vi "Calculate Index Array.vi"(8 "error in (no error)":errorcluster, 10 "3D Waterfall Datatype.lvclass in":refnum<class "3D Waterfall Datatype.lvclass">, 11 "Plot Representation In":T1) -> (0 "error out":errorcluster, 2 "3D Waterfall Datatype.lvclass out":refnum<class "3D Waterfall Datatype.lvclass">, 3 "Plot Representation Out":T1)   [LabVIEW 2017, in "3D Waterfall Datatype.lvclass"]
uses:
  <vilib>/Math Plots/3D Math Plots/3D Waterfall/3D Waterfall Datatype/3D Waterfall Datatype.lvclass
  <vilib>/Math Plots/3D Math Plots/3D Plot/3D Plot/Typedef/Plot Representation.ctl
  <vilib>/Math Plots/3D Math Plots/3D Plot/3D Plot/Typedef/Range Clusters.ctl
  <vilib>/Math Plots/3D Math Plots/3D Plot/3D Plot/Typedef/Mesh Data.ctl
  <vilib>/Math Plots/3D Math Plots/3D Plot/3D Plot/3D Plot.lvclass
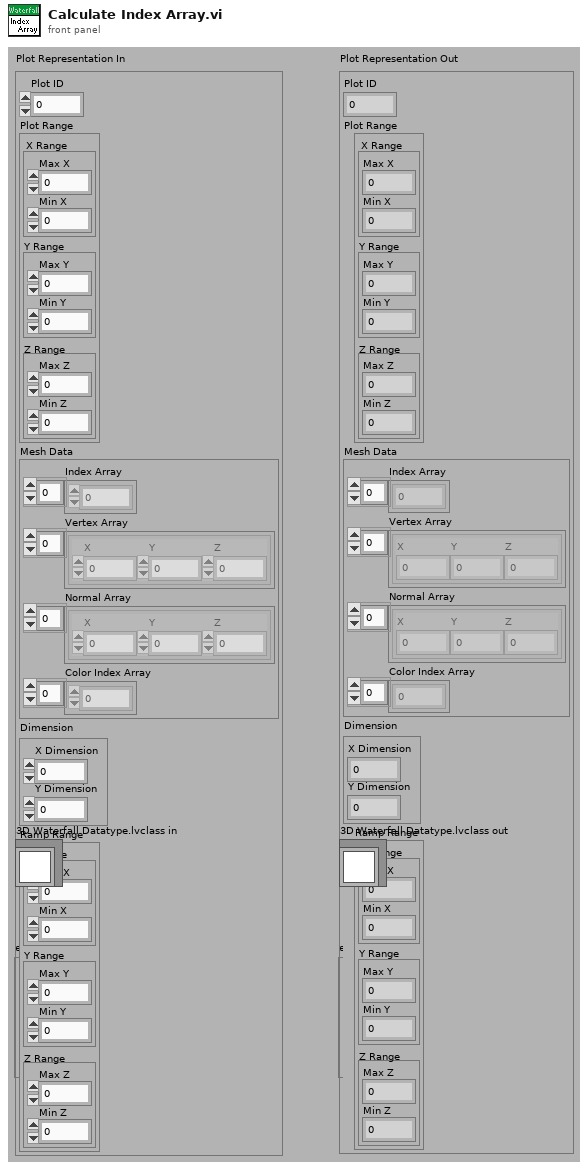
[diagram p1: front panel]
types:
  T1 = typedef "3D Plot.lvclass/Plot Representation.ctl" = cluster{"Plot ID":i32, "Plot Range":T2, "Mesh Data":T3, "Dimension":cluster{"X Dimension":i32, "Y Dimension":i32}, "Ramp Range":T2}
  T2 = typedef "3D Plot.lvclass/Range Clusters.ctl" = cluster{"X Range":cluster{"Max X":sgl, "Min X":sgl}, "Y Range":cluster{"Max Y":sgl, "Min Y":sgl}, "Z Range":cluster{"Max Z":sgl, "Min Z":sgl}}
  T3 = typedef "3D Plot.lvclass/Mesh Data.ctl" = cluster{"Index Array":u32[], "Vertex Array":cluster{"X":sgl, "Y":sgl, "Z":sgl}[], "Normal Array":cluster{"X":sgl, "Y":sgl, "Z":sgl}[], "Color Index Array":i32[]}
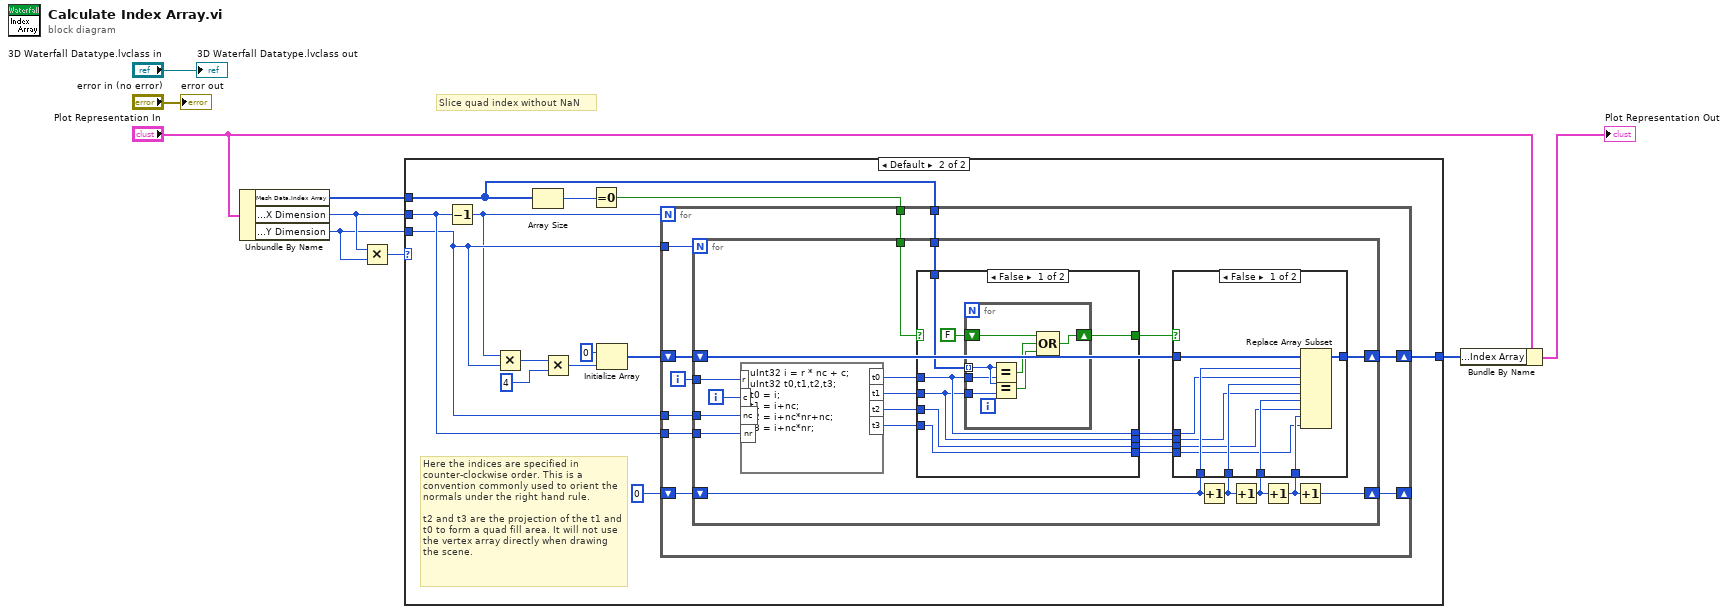
[diagram p0: block diagram]
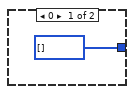
[diagram p2: hidden frame]
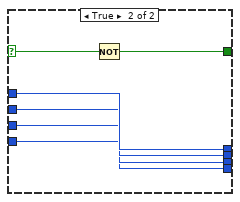
[diagram p4: hidden frame]
diagram:
  # "Slice quad index without NaN"
  n1 = Unbundle By Name("Plot Representation In") -> ("Mesh Data.Index Array"=w1:u32[], "Dimension.X Dimension"=w4:i32, "Dimension.Y Dimension"=w3:i32)
  n2 = Multiply(x=w4, y=w3) -> (x*y=w2:i32)
  n3 = case shown="Default" w2 {
    tunnel: [u32[] [] w23] -> w5
    tunnel: w4 -> [_ w17]
    tunnel: w3 -> [_ w16]
    tunnel: w1 -> [_ w12]
    frame 0 {
    }
    frame Default {
      # "Here the indices are specified in counter-clockwise order. This is a convention commonly used to orient the normals under the right hand rule.\n\nt2 and t3 are the projection of the t1 and t0 to form a quad fill area. It will not use the vertex array directly when drawing the scene."
      n4 = Decrement(x=w17) -> (x-1=w14:i32)
      n5 = Multiply(x=w14, y=w16) -> (x*y=w20:i32)
      n6 = Array Size(array=w12) -> (size(s)=w13:i32)
      n7 = Multiply(x=w20, y=4) -> (x*y=w22:i32)
      n8 = Equal To 0?(x=w13) -> (x = 0?=w11:bool)
      n9 = Initialize Array(u32 0, w22) -> (w18:u32[])
      n10 = for {
        N: w14 -> [_]
        shift-right: [w29] -> w23
        shift-left: w18 -> [w33]
        tunnel: w16 -> [w31]
        tunnel: w16 -> [w30]
        tunnel: w17 -> [w28]
        shift-right: [w27] -> _
        shift-left: 0 -> [w26]
        tunnel: w12 -> [w25]
        tunnel: w11 -> [w24]
        i -> [w32]
        n11 = for {
          N: w31 -> [_]
          tunnel: w32 -> [w55]
          tunnel: w30 -> [w53]
          shift-right: [w49] -> w29
          shift-left: w33 -> [w50]
          tunnel: w28 -> [w52]
          shift-right: [w51] -> w27
          shift-left: w26 -> [w45]
          tunnel: w25 -> [w44]
          tunnel: w24 -> [w43]
          i -> [w54]
          n12 = formula code="uInt32 i = r * nc + c; \nuInt32 t0,t1,t2,t3;\nt0 = i; \nt1 = i+nc; \nt2 = i+nc*nr+nc; \nt3 = i+nc*nr;"("r"=w55, "nc"=w53, "c"=w54, "nr"=w52) -> ("t0"=w42:u32, "t1"=w41:u32, "t2"=w40:u32, "t3"=w39:u32)
          n13 = case shown="False" w43 {
            selector: w43 -> [_ w82]
            tunnel: [w70 w86] -> w38
            tunnel: w42 -> [w70 w86]
            tunnel: [w69 w85] -> w37
            tunnel: w41 -> [w69 w85]
            tunnel: [w68 w84] -> w36
            tunnel: w40 -> [w68 w84]
            tunnel: [w67 w83] -> w35
            tunnel: w39 -> [w67 w83]
            tunnel: w44 -> [w73 _]
            tunnel: [w71 w81] -> w34
            frame False {
              n14 = for {
                tunnel: w73 -> [w80] mode=indexing
                tunnel: w70 -> [w79]
                tunnel: w69 -> [w74]
                shift-right: [w76] -> w71
                shift-left: FALSE -> [w75]
                n15 = Equal?(x=w80, y=w79) -> (x = y?=w78:bool)
                n16 = Equal?(x=w80, y=w74) -> (x = y?=w77:bool)
                n17 = Compound Arithmetic op=OR(w75, w78, w77) -> (w76:bool)
              }
            }
            frame True {
              n18 = Not(x=w82) -> (.not. x?=w81:bool)
            }
          }
          n19 = Increment(x=w45) -> (x+1=w46:i32)
          n20 = Increment(x=w46) -> (x+1=w47:i32)
          n21 = Increment(x=w47) -> (x+1=w48:i32)
          n22 = case shown="False" w34 {
            tunnel: w50 -> [w65 w66]
            tunnel: [w64 w66] -> w49
            tunnel: w48 -> [w63 _]
            tunnel: w47 -> [w62 _]
            tunnel: w46 -> [w61 _]
            tunnel: w45 -> [w60 _]
            tunnel: w38 -> [w59 _]
            tunnel: w37 -> [w58 _]
            tunnel: w36 -> [w57 _]
            tunnel: w35 -> [w56 _]
            frame False {
              n23 = Replace Array Subset(array=w65, new element #1=w59, index #1=w60, new element #2=w58, index #2=w61, new element #3=w57, index #3=w62, new element #4=w56, index #4=w63) -> (w64:u32[])
            }
            frame True {
            }
          }
          n24 = Increment(x=w48) -> (x+1=w51:i32)
        }
      }
    }
  }
  n25 = Bundle By Name(cluster="Plot Representation In", "Mesh Data.Index Array"=w5) -> (→"Plot Representation Out":T1)
  "error out" <- "error in (no error)"
  "3D Waterfall Datatype.lvclass out" <- "3D Waterfall Datatype.lvclass in"
